vi "Copy and Rename lvlib.vi"(8 "error in":errorcluster, 9 "New lvlib Name":string, 10 "Destination Directory Path":path, 11 "lvlib Path":path) -> (0 "error out":errorcluster, 3 "New Library Path":path)   [LabVIEW 2026, in "NIVS_CDEW_MetaDataObj.lvclass"]
uses:
  NIVS_CDEW_MetaDataObj.lvclass
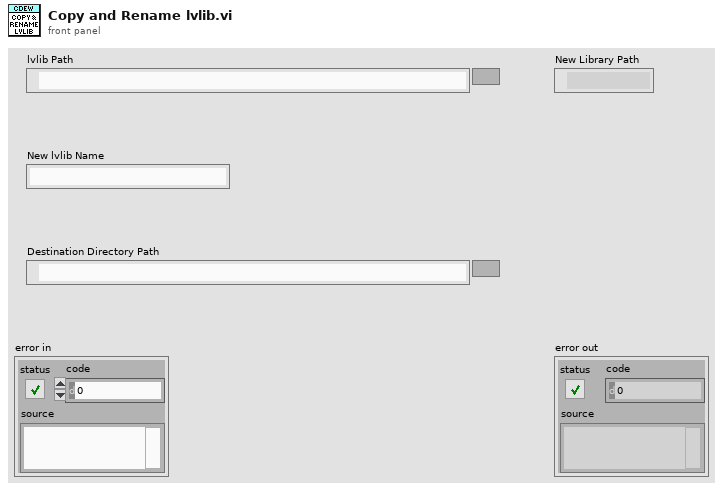
[diagram p1: front panel]
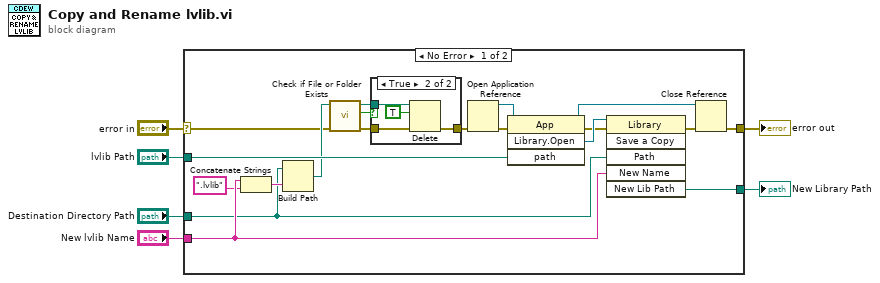
[diagram p0: block diagram]
diagram:
  n1 = case shown="No Error" "error in" {
    selector: "error in" -> [w9 w31]
    tunnel: "lvlib Path" -> [w23 _]
    tunnel: "Destination Directory Path" -> [w7 _]
    tunnel: "New lvlib Name" -> [w17 _]
    tunnel: [w20 w31] -> w3
    tunnel: [w19 _] -> w2
    frame No Error {
      n2 = Concatenate Strings(w17, ".lvlib" ("string")) -> (w15:string)
      n3 = Build Path(base path=w7, name or relative path=w15) -> (appended path=w14:path)
      n4 = call <vilib>:"Check if File or Folder Exists.vi"("error in (no error)"=w9, "path"=w14) -> ("error out"=w11:errorcluster, "file or folder exists?"=w13:bool, "dup path"=w12:path)  [unwired: 7 in]
      n5 = case shown="True" w13 {
        tunnel: w12 -> [_ w30]
        tunnel: w11 -> [w26 w29]
        tunnel: [w26 w27] -> w8
        frame False {
        }
        frame True {
          n6 = Delete(path (use dialog)=w30, entire hierarchy (F)=TRUE, error in=w29) -> (error out=w27:errorcluster)  [unwired: 2 in, 2 out]
        }
      }
      n7 = Open Application Reference(8:w8) -> (0:w24:errorcluster, 3:w25:refnum<vi>)  [unwired: 3 in]
      n8 = invoke class="App" method="Library.Open"(reference=w25, error in=w24, "path"=w23) -> (reference out=w21:refnum<vi>, error out=w10:errorcluster, "Open Library"=w18:refnum<vi>)  [unwired: 1 in, 1 out]
      n9 = invoke class="Library" method="Save a Copy"(reference=w18, error in=w10, "Path"=w7, "New Name"=w17) -> (error out=w22:errorcluster, "New Lib Path"=w19:path)  [unwired: 2 in, 4 out]
      n10 = Close Reference(reference=w21, error in (no error)=w22) -> (error out=w20:errorcluster)
    }
    frame Error {
    }
  }
  "error out" <- w3
  "New Library Path" <- w2
